vi "Read Execution Error.vi"(8 "error in (no error)":errorcluster, 11 "VISA resource name":refnum<visa-resource-name>) -> (0 "error out":errorcluster, 1 "Error Message":string, 2 "Error Code":i32, 3 "VISA resource name out":refnum<visa-resource-name>)   [LabVIEW 2018, in "LeCroy Wave Series.lvlib"]
doc: "Reads and clears the contents of the Execution error Register (EXR). The EXR register specifies the type of the last error detected during execution."
uses:
  LeCroy Wave Series.lvlib
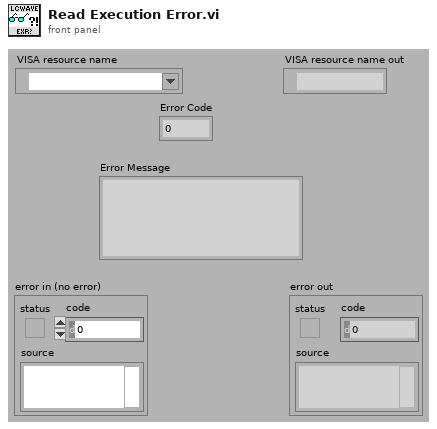
[diagram p1: front panel]
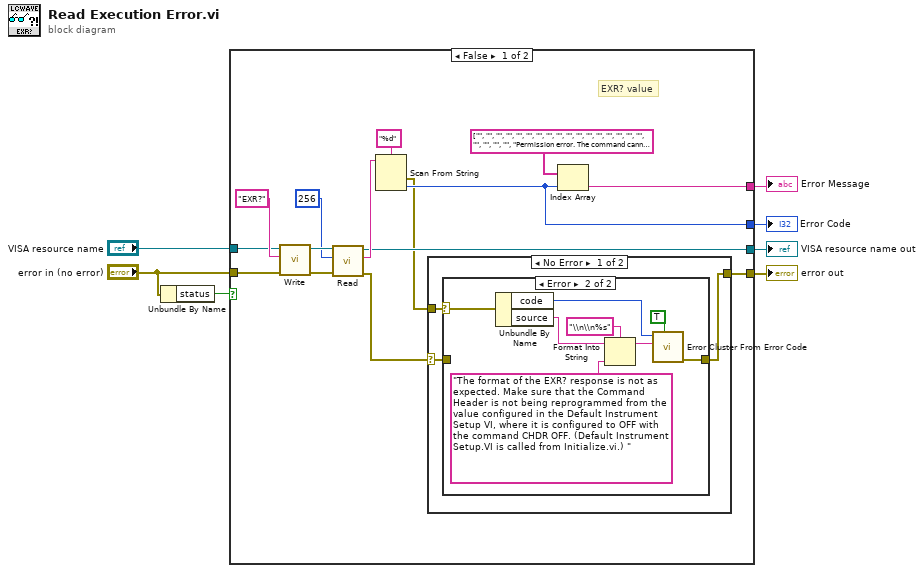
[diagram p0: block diagram]
diagram:
  n1 = Unbundle By Name("error in (no error)") -> ("status"=w1:bool)
  n2 = case shown="False" w1 {
    tunnel: [w16 _] -> w7
    tunnel: "VISA resource name" -> [w15 w37]
    tunnel: "error in (no error)" -> [w14 w36]
    tunnel: [w13 w37] -> w5
    tunnel: [w8 w36] -> w4
    tunnel: [w12 _] -> w3
    frame False {
      # "EXR? value"
      n3 = call "Write.vi"("error in (no error)"=w14, "Write Buffer"="EXR?" ("write buffer"), "VISA resource name"=w15) -> ("error out"=w21:errorcluster, "VISA resource name out"=w22:refnum<visa-resource-name>)  [unwired: 7 in]
      n4 = call "Read.vi"("error in (no error)"=w21, "Byte Count"=u32 256 ("byte count"), "VISA resource name"=w22) -> ("error out"=w9:errorcluster, "Read Buffer"=w18:string, "VISA resource name out"=w13:refnum<visa-resource-name>)  [unwired: 5 in, 1 out]
      n5 = Scan From String(format string="%d", input string=w18) -> (error out=w10:errorcluster, output 1=w16:i32)  [unwired: 3 in, 2 out]
      n6 = case shown="No Error" w9 {
        selector: w9 -> [w25 w35]
        tunnel: [w24 w35] -> w8
        tunnel: w10 -> [w23 _]
        frame No Error {
          n7 = case shown="Error" w23 {
            selector: w23 -> [_ w30]
            tunnel: w25 -> [w26 _]
            tunnel: [w26 w33] -> w24
            frame No Error {
            }
            frame Error {
              n8 = Unbundle By Name(w30) -> ("code"=w29:i32, "source"=w28:string)
              n9 = Format Into String(format string="\\n\\n%s", initial string=w28, "The format of the EXR? response is not as expected. Make sure that the Command Header is not being reprogrammed from the value configured in the Default Instrument Setup VI, where it is configured to OFF with the command CHDR OFF. (Default Instrument Setup.VI is called from Initialize.vi.) " ("source")) -> (resulting string=w27:string)  [unwired: 1 in, 1 out]
              n10 = call <vilib>:"Error Cluster From Error Code.vi"("show call chain? (False)"=TRUE, "error message (\"\")"=w27, "error code (0)"=w29) -> ("error out"=w33:errorcluster)  [unwired: 6 in]
            }
          }
        }
        frame Error {
        }
      }
      n11 = Index Array(array=string[] ["", "", "", "", "", "", "", "", "", "", "", "", "", "", "", "", "", "", "", "", "", "Permission error. The command cannot be executed in local mode.", "Environment error. The oscilloscope is not configured to correctly process a command. For instance, the oscilloscope cannot be set to RIS at a slow timebase.", "Option error. The command applies to an option which has not been installed.", "Unresolved parsing error.", "Parameter error. Too many parameters specified.", "Non-implemented command.", "Parameter missing. A parameter was expected by the command.", "", "", "Hex data error. A non-hexadecimal character has been detected in a hex data block.", "Waveform error. The amount of data received does not correspond to descriptor indicators.", "Waveform descriptor error. An invalid waveform descriptor has been detected.", "Waveform text error. A corrupted waveform user text has been detected.", "Waveform time error. Invalid RIS or TRIG time data has been detected.", "Waveform data error. Invalid waveform data have been detected.", "Panel setup error. An invalid panel setup data block has been detected.", "", "", "", "", "", "", "", "", "", "", "", "", "", "No mass storage present when user attempted to access it. *", "Mass storage not formatted when user attempted to access it. *", "", "Mass storage was write protected when user attempted to create a file, to delete a file, or to format the device. *", "Bad mass storage detected during formatting. *", "Mass storage root directory full. Cannot add directory. *", "Mass storage full when user attempted to write to it. *", "Mass storage file sequence numbers exhausted (999 reached). *", "Mass storage file not found. *", "Requested directory not found. *", "", "Mass storage filename not DOS compatible, or illegal filename. *", "Cannot write on mass storage because filename already exists. *"], index=w16) -> (element=w12:string)
    }
    frame True {
    }
  }
  "VISA resource name out" <- w5
  "error out" <- w4
  "Error Message" <- w3
  "Error Code" <- w7
